vi "Axis Mirorred.vi"(4 "Character Size":sgl=0.5, 5 "Half plane?":bool=TRUE, 6 "Axis label?":bool, 7 "Color":T1={"Red"=1.0, "Green"=0.0, "Blue"=0.0, "Alpha"=1.0}, 8 "error in (no error)":errorcluster, 9 "Radius":sgl=0.01, 10 "Length":sgl=2.0) -> (0 "error out":errorcluster, 3 "New Object Refnum":refnum<vi>)   [LabVIEW 2021]
uses:
  <vilib>/Utility/miscctls.llb/LVSceneTextAlignment.ctl
  <vilib>/picture/3D Picture Control/Object/Create Object (name).vi
  <vilib>/picture/3D Picture Control/Object/Create Object (drawable).vi
  <vilib>/picture/3D Picture Control/Object/Add Object (no reference).vi
  <vilib>/picture/3D Picture Control/NI_3D Picture Control.lvlib
panel:
  in  "Name":string="XYZ axis"
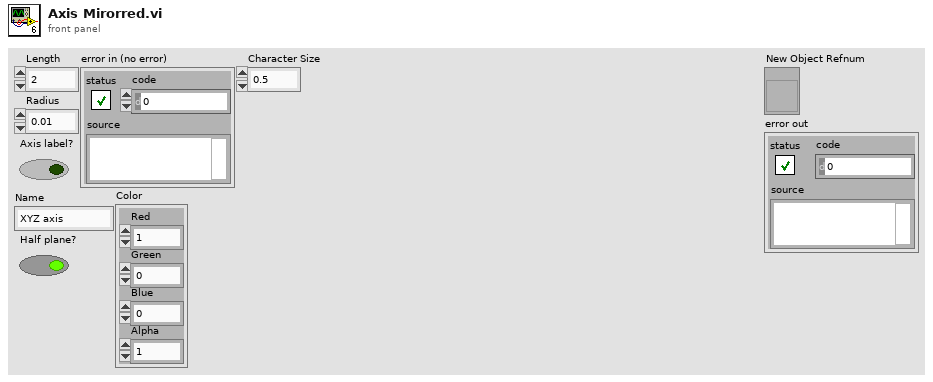
[diagram p1: front panel]
types:
  T1 = cluster{"Red":sgl, "Green":sgl, "Blue":sgl, "Alpha":sgl}
  T2 = typedef "LVSceneTextAlignment.ctl" = cluster{"Horizontal Alignment":enum8{"Left", "Right", "Center"}, "Vertical Alignment":enum8{"Top", "Bottom", "Center", "Base Line", "Bottom Base Line"}}
  T3 = cluster{"Alignment":T2, "Axis Alignment":enum8{"X-Y", "Y-Z", "X-Z", "Reversed X-Y", "Reversed Y-Z", "Reversed X-Z", "Screen"}, "Vertical?":bool, "Wrap Distance":sgl}
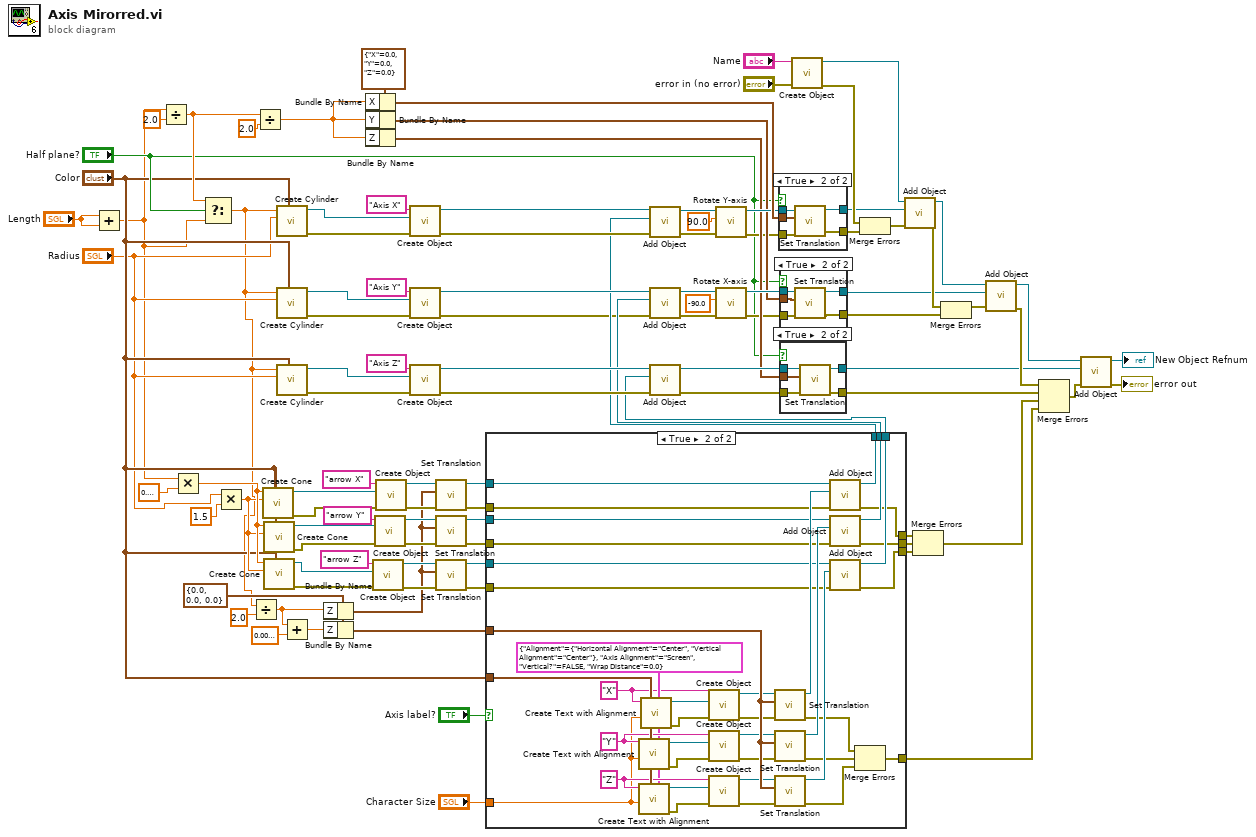
[diagram p0: block diagram]
diagram:
  w50 = cluster{"X":sgl, "Y":sgl, "Z":sgl} {"X"=0.0, "Y"=0.0, "Z"=0.0} ("Translation")
  w35 = cluster{"X":sgl, "Y":sgl, "Z":sgl} {"X"=0.0, "Y"=0.0, "Z"=0.0} ("Translation")
  n1 = Add(x="Length", y="Length") -> (x+y=w2:sgl)
  n2 = Divide(x=w2, y=sgl 2.0) -> (x/y=w71:sgl)
  n3 = Multiply(x=w2, y=sgl 0.1) -> (x*y=w13:sgl)
  n4 = Select(t=w71, s="Half plane?", f=w2) -> (s? t:f=w1:sgl)
  n5 = Multiply(x="Radius", y=sgl 1.5) -> (x*y=w12:sgl)
  n6 = Divide(x=w1, y=sgl 2.0 ("x")) -> (x/y=w14:sgl)
  n7 = Divide(x=w71, y=sgl 2.0) -> (x/y=w49:sgl)
  n8 = call <vilib>:"Create Cone.vi"("Color"="Color", "Radius"=w12, "Height"=w13) -> ("error out"=w15:errorcluster, "New Cone Refnum"=w57:refnum<vi>)  [unwired: 7 in]
  n9 = call <vilib>:"Create Cone.vi"("Color"="Color", "Radius"=w12, "Height"=w13) -> ("error out"=w7:errorcluster, "New Cone Refnum"=w9:refnum<vi>)  [unwired: 7 in]
  n10 = call <vilib>:"Create Cone.vi"("Color"="Color", "Radius"=w12, "Height"=w13) -> ("error out"=w8:errorcluster, "New Cone Refnum"=w10:refnum<vi>)  [unwired: 7 in]
  n11 = call <vilib>:"Create Cylinder.vi"("Color"="Color", "Radius"="Radius", "Height"=w1) -> ("error out"=w87:errorcluster, "New Cylinder Refnum"=w93:refnum<vi>)  [unwired: 7 in]
  n12 = call <vilib>:"Create Cylinder.vi"("Color"="Color", "Radius"="Radius", "Height"=w1) -> ("error out"=w86:errorcluster, "New Cylinder Refnum"=w95:refnum<vi>)  [unwired: 7 in]
  n13 = call <vilib>:"Create Cylinder.vi"("Color"="Color", "Radius"="Radius", "Height"=w1) -> ("error out"=w85:errorcluster, "New Cylinder Refnum"=w94:refnum<vi>)  [unwired: 7 in]
  n14 = Add(x=w14, y=sgl 0.01) -> (x+y=w26:sgl)
  n15 = Bundle By Name(cluster=w35, "Z"=w14) -> (w46:cluster{"X":sgl, "Y":sgl, "Z":sgl})
  n16 = Bundle By Name(cluster=w35, "Z"=w26) -> (w31:cluster{"X":sgl, "Y":sgl, "Z":sgl})
  n17 = Bundle By Name(cluster=w50, "X"=w49) -> (w73:cluster{"X":sgl, "Y":sgl, "Z":sgl})
  n18 = Bundle By Name(cluster=w50, "Y"=w49) -> (w51:cluster{"X":sgl, "Y":sgl, "Z":sgl})
  n19 = Bundle By Name(cluster=w50, "Z"=w49) -> (w48:cluster{"X":sgl, "Y":sgl, "Z":sgl})
  n20 = call-poly <vilib>:"Create Object.vi"("error in (no error)"=w8, "Geometry"=w10, "Name"="arrow Z") -> ("error out"=w58:errorcluster, "Scene:New Object"=w59:refnum<vi>)  [unwired: 7 in]
  n21 = call-poly <vilib>:"Create Object.vi"("error in (no error)"=w7, "Geometry"=w9, "Name"="arrow Y") -> ("error out"=w63:errorcluster, "Scene:New Object"=w62:refnum<vi>)  [unwired: 7 in]
  n22 = call-poly <vilib>:"Create Object.vi"("error in (no error)"=w15, "Geometry"=w57, "Name"="arrow X") -> ("error out"=w76:errorcluster, "Scene:New Object"=w77:refnum<vi>)  [unwired: 7 in]
  n23 = call-poly <vilib>:"Create Object.vi"("error in (no error)"=w87, "Geometry"=w93, "Name"="Axis X") -> ("error out"=w41:errorcluster, "Scene:New Object"=w66:refnum<vi>)  [unwired: 7 in]
  n24 = call-poly <vilib>:"Create Object.vi"("error in (no error)"=w86, "Geometry"=w95, "Name"="Axis Y") -> ("error out"=w18:errorcluster, "Scene:New Object"=w61:refnum<vi>)  [unwired: 7 in]
  n25 = call-poly <vilib>:"Create Object.vi"("error in (no error)"=w85, "Geometry"=w94, "Name"="Axis Z") -> ("error out"=w45:errorcluster, "Scene:New Object"=w56:refnum<vi>)  [unwired: 7 in]
  n26 = call <vilib>:"Set Translation.vi"("error in (no error)"=w76, "Translation"=w46, "Scene Object"=w77) -> ("error out"=w25:errorcluster, "Translated Object"=w37:refnum<vi>)  [unwired: 7 in]
  n27 = call <vilib>:"Set Translation.vi"("error in (no error)"=w63, "Translation"=w46, "Scene Object"=w62) -> ("error out"=w24:errorcluster, "Translated Object"=w34:refnum<vi>)  [unwired: 7 in]
  n28 = call <vilib>:"Set Translation.vi"("error in (no error)"=w58, "Translation"=w46, "Scene Object"=w59) -> ("error out"=w27:errorcluster, "Translated Object"=w32:refnum<vi>)  [unwired: 7 in]
  n29 = case shown="True" "Axis label?" {
    tunnel: w37 -> [w108 w145]
    tunnel: [w108 w144] -> w36
    tunnel: w34 -> [w107 w143]
    tunnel: [w107 w141] -> w33
    tunnel: w32 -> [w103 w140]
    tunnel: w31 -> [_ w139]
    tunnel: [w103 w137] -> w30
    tunnel: w27 -> [w105 w136]
    tunnel: w25 -> [w106 w135]
    tunnel: w24 -> [w104 w134]
    tunnel: [w106 w133] -> w23
    tunnel: [w104 w132] -> w22
    tunnel: [w105 w131] -> w21
    tunnel: [_ w130] -> w19
    tunnel: "Color" -> [_ w129]
    tunnel: "Character Size" -> [_ w109]
    frame False {
    }
    frame True {
      w121 = "Z" ("text")
      w126 = "Y" ("text")
      w116 = T3 {"Alignment"={"Horizontal Alignment"=enum."Center", "Vertical Alignment"=enum."Center"}, "Axis Alignment"=enum."Screen", "Vertical?"=FALSE, "Wrap Distance"=0.0} ("Font options")
      w114 = "X" ("text")
      n30 = call <vilib>:"Create Text with Alignment.vi"("Font Options"=w116, "Color"=w129, "Character Size"=w109, "Text"=w126) -> ("error out"=w118:errorcluster, "New Text Refnum"=w125:refnum<vi>)  [unwired: 6 in]
      n31 = call <vilib>:"Create Text with Alignment.vi"("Font Options"=w116, "Color"=w129, "Character Size"=w109, "Text"=w121) -> ("error out"=w120:errorcluster, "New Text Refnum"=w122:refnum<vi>)  [unwired: 6 in]
      n32 = call <vilib>:"Create Text with Alignment.vi"("Font Options"=w116, "Color"=w129, "Character Size"=w109, "Text"=w114) -> ("error out"=w113:errorcluster, "New Text Refnum"=w128:refnum<vi>)  [unwired: 6 in]
      n33 = call-poly <vilib>:"Create Object.vi"("error in (no error)"=w113, "Geometry"=w128, "Name"=w114) -> ("error out"=w115:errorcluster, "Scene:New Object"=w127:refnum<vi>)  [unwired: 7 in]
      n34 = call-poly <vilib>:"Create Object.vi"("error in (no error)"=w118, "Geometry"=w125, "Name"=w126) -> ("error out"=w117:errorcluster, "Scene:New Object"=w124:refnum<vi>)  [unwired: 7 in]
      n35 = call-poly <vilib>:"Create Object.vi"("error in (no error)"=w120, "Geometry"=w122, "Name"=w121) -> ("error out"=w119:errorcluster, "Scene:New Object"=w123:refnum<vi>)  [unwired: 7 in]
      n36 = call <vilib>:"Set Translation.vi"("error in (no error)"=w115, "Translation"=w139, "Scene Object"=w127) -> ("error out"=w110:errorcluster, "Translated Object"=w146:refnum<vi>)  [unwired: 7 in]
      n37 = call <vilib>:"Set Translation.vi"("error in (no error)"=w117, "Translation"=w139, "Scene Object"=w124) -> ("error out"=w111:errorcluster, "Translated Object"=w142:refnum<vi>)  [unwired: 7 in]
      n38 = call <vilib>:"Set Translation.vi"("error in (no error)"=w119, "Translation"=w139, "Scene Object"=w123) -> ("error out"=w112:errorcluster, "Translated Object"=w138:refnum<vi>)  [unwired: 7 in]
      n39 = call-poly <vilib>:"Add Object.vi"("error in (no error)"=w135, "New Object In"=w146, "Scene Object In"=w145) -> ("error out"=w133:errorcluster, "Scene Object Out"=w144:refnum<vi>)  [unwired: 7 in]
      n40 = call-poly <vilib>:"Add Object.vi"("error in (no error)"=w134, "New Object In"=w142, "Scene Object In"=w143) -> ("error out"=w132:errorcluster, "Scene Object Out"=w141:refnum<vi>)  [unwired: 7 in]
      n41 = call-poly <vilib>:"Add Object.vi"("error in (no error)"=w136, "New Object In"=w138, "Scene Object In"=w140) -> ("error out"=w131:errorcluster, "Scene Object Out"=w137:refnum<vi>)  [unwired: 7 in]
      n42 = Merge Errors(w110, w111, w112) -> (w130:errorcluster)
    }
  }
  n43 = call-poly <vilib>:"Add Object.vi"("error in (no error)"=w41, "New Object In"=w36, "Scene Object In"=w66) -> ("error out"=w40:errorcluster, "Scene Object Out"=w65:refnum<vi>)  [unwired: 7 in]
  n44 = call-poly <vilib>:"Add Object.vi"("error in (no error)"=w18, "New Object In"=w33, "Scene Object In"=w61) -> ("error out"=w17:errorcluster, "Scene Object Out"=w60:refnum<vi>)  [unwired: 7 in]
  n45 = call-poly <vilib>:"Add Object.vi"("error in (no error)"=w45, "New Object In"=w30, "Scene Object In"=w56) -> ("error out"=w44:errorcluster, "Scene Object Out"=w53:refnum<vi>)  [unwired: 7 in]
  n46 = call <vilib>:"Rotate Y-axis.vi"("error in (no error)"=w40, "angle"=90.0, "Scene Object In"=w65) -> ("error out"=w39:errorcluster, "Scene Object Out"=w70:refnum<vi>)  [unwired: 7 in]
  n47 = call <vilib>:"Rotate X-axis.vi"("error in (no error)"=w17, "angle"=-90.0, "Scene Object In"=w60) -> ("error out"=w42:errorcluster, "Scene Object Out"=w55:refnum<vi>)  [unwired: 7 in]
  n48 = case shown="True" "Half plane?" {
    tunnel: w70 -> [w148 w153]
    tunnel: w73 -> [_ w152]
    tunnel: [w148 w151] -> w69
    tunnel: [w147 w150] -> w68
    tunnel: w39 -> [w147 w149]
    frame False {
    }
    frame True {
      n49 = call <vilib>:"Set Translation.vi"("error in (no error)"=w149, "Translation"=w152, "Scene Object"=w153) -> ("error out"=w150:errorcluster, "Translated Object"=w151:refnum<vi>)  [unwired: 7 in]
    }
  }
  n50 = case shown="True" "Half plane?" {
    tunnel: w55 -> [w155 w160]
    tunnel: [w155 w159] -> w54
    tunnel: [w154 w158] -> w47
    tunnel: w51 -> [_ w157]
    tunnel: w42 -> [w154 w156]
    frame False {
    }
    frame True {
      n51 = call <vilib>:"Set Translation.vi"("error in (no error)"=w156, "Translation"=w157, "Scene Object"=w160) -> ("error out"=w158:errorcluster, "Translated Object"=w159:refnum<vi>)  [unwired: 7 in]
    }
  }
  n52 = case shown="True" "Half plane?" {
    tunnel: w53 -> [w162 w167]
    tunnel: [w162 w166] -> w52
    tunnel: [w161 w165] -> w43
    tunnel: w48 -> [_ w164]
    tunnel: w44 -> [w161 w163]
    frame False {
    }
    frame True {
      n53 = call <vilib>:"Set Translation.vi"("error in (no error)"=w163, "Translation"=w164, "Scene Object"=w167) -> ("error out"=w165:errorcluster, "Translated Object"=w166:refnum<vi>)  [unwired: 7 in]
    }
  }
  n54 = call-poly <vilib>:"Create Object.vi"("error in (no error)"="error in (no error)", "Name"="Name") -> ("error out"=w84:errorcluster, "Scene:New Object"=w101:refnum<vi>)  [unwired: 8 in]
  n55 = Merge Errors(w84, w68) -> (w83:errorcluster)
  n56 = call-poly <vilib>:"Add Object.vi"("error in (no error)"=w83, "New Object In"=w69, "Scene Object In"=w101) -> ("error out"=w82:errorcluster, "Scene Object Out"=w100:refnum<vi>)  [unwired: 7 in]
  n57 = Merge Errors(w23, w22, w21) -> (w20:errorcluster)
  n58 = Merge Errors(w82, w47) -> (w81:errorcluster)
  n59 = call-poly <vilib>:"Add Object.vi"("error in (no error)"=w81, "New Object In"=w54, "Scene Object In"=w100) -> ("error out"=w80:errorcluster, "Scene Object Out"=w99:refnum<vi>)  [unwired: 7 in]
  n60 = Merge Errors(w80, w43, w20, w19) -> (w79:errorcluster)
  n61 = call-poly <vilib>:"Add Object.vi"("error in (no error)"=w79, "New Object In"=w52, "Scene Object In"=w99) -> ("error out"=→"error out":errorcluster, "Scene Object Out"=→"New Object Refnum":refnum<vi>)  [unwired: 7 in]
